vi "FTW-Example-Service-Launch.vi"(0 "Number":u32, 9 "Timeout":i32=1000 format="%dmsec", 11 "error in":errorcluster) -> (4 "FTW Actor Connector":refnum<class "FTW-Example-Service.lvclass">, 6 "Initialized Response":string, 8 "Instance Inbox Address":string, 15 "error out":errorcluster)   [LabVIEW 2013, in "FTW-Example-Service.lvclass"]
uses:
  FTW-Example-Service.lvclass
  source/actor/Connector/FTW-ActorConnector.lvclass
  Core/FTW-Example-Service-Core.lvclass
panel:
  in  "Service Name":string
  in  "Boolean":bool
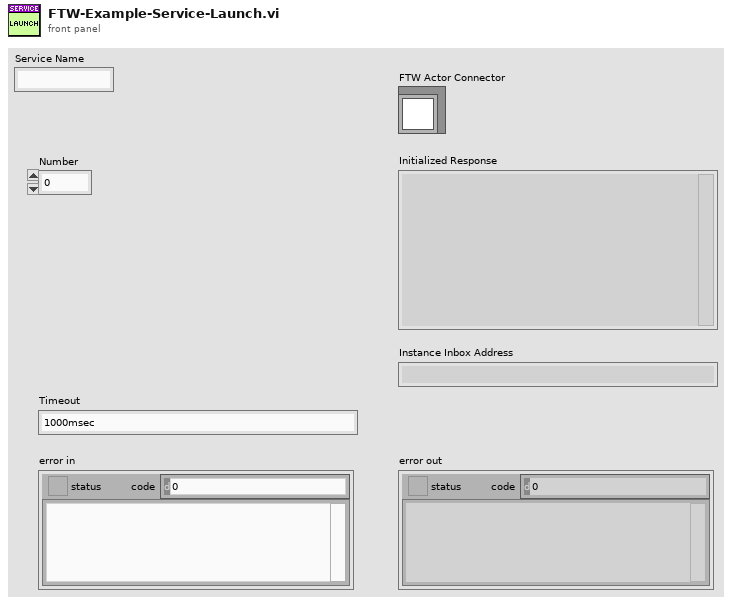
[diagram p1: front panel]
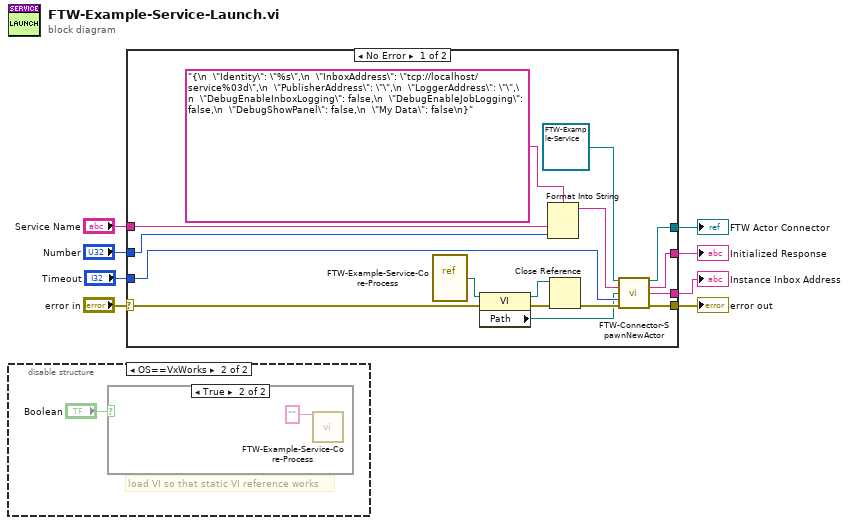
[diagram p0: block diagram]
diagram:
  n1 = disable-structure shown="OS==VxWorks" {
    frame condition #0 (active) {
    }
    frame condition #1 {
      # "load VI so that static VI reference works"
      n2 = case shown="True" "Boolean" {
        frame False {
        }
        frame True {
          n3 = call "FTW-Example-Service-Core-Process.vi"("FTW Actor Instance Configuration"="") -> ()  [unwired: 14 in, 1 out]
        }
      }
    }
  }
  n4 = case shown="No Error" "error in" {
    selector: "error in" -> [w17 w27]
    tunnel: [w25 w27] -> w8
    tunnel: [w24 _] -> w7
    tunnel: "Timeout" -> [w23 _]
    tunnel: [w22 _] -> w5
    tunnel: [w21 _] -> w4
    tunnel: "Number" -> [w12 _]
    tunnel: "Service Name" -> [w11 _]
    frame No Error {
      n5 = vi-ref "FTW-Example-Service-Core-Process.vi"() -> (w20:refnum<vi>)
      n6 = property class="VI"(reference=w20, error in=w17) -> (reference out=w19:refnum<vi>, error out=w18:errorcluster, "Path"=w15:path)
      n7 = Format Into String(format string="{\n  \"Identity\": \"%s\",\n  \"InboxAddress\": \"tcp://localhost/service%03d\",\n  \"PublisherAddress\": \"\",\n  \"LoggerAddress\": \"\",\n  \"DebugEnableInboxLogging\": false,\n  \"DebugEnableJobLogging\": false,\n  \"DebugShowPanel\": false,\n  \"My Data\": false\n}" ("Configuration"), w11, w12) -> (resulting string=w13:string)  [unwired: 2 in, 1 out]
      n8 = Close Reference(reference=w19, error in (no error)=w18) -> (error out=w16:errorcluster)
      n9 = call "FTW-Connector-SpawnNewActor.vi"("FTW Actor Connector Type"=refnum<class "FTW-Example-Service.lvclass"> refnum ("TTK_Splashscreen.lvclass"), "Configuration"=w13, "Actor VI Filepath"=w15, "Timeout"=w23, "error in"=w16) -> ("FTW Actor Connector"=w24:refnum<class "FTW-Example-Service.lvclass">, "Initialized Response"=w22:string, "Instance Inbox Address"=w21:string, "error out"=w25:errorcluster)  [unwired: 6 in, 1 out]
    }
    frame Error {
    }
  }
  "error out" <- w8
  "FTW Actor Connector" <- w7
  "Initialized Response" <- w5
  "Instance Inbox Address" <- w4
